vi "0716206_clock.vi"() -> ()   [LabVIEW 2021]
uses:
  <vilib>/Utility/miscctls.llb/LVPositionTypeDef.ctl
  <vilib>/Analysis/NI_AALBase.lvlib
panel:
  in  "Alarm Sound Path":path
  in  "Dial":dbl(knob) scale=0.0..1440.0
  in  "Set Time":bool
  out "Alarm Info.":string
  out "Sound Is Playing?":bool
  in  "Stop 2":bool
  in  "Sound Device ID":u32
  out "Alarm ring":bool=TRUE
  out "String 2":string
  out "String":string
  in  "Enable Alarm":bool
  in  "m0":bool
  in  "m1":bool
  in  "m2":bool
  in  "m3":bool
  in  "m4":bool
  in  "m5":bool
  out "alarm_min2":dbl
  in  "alarm_am":bool
  out "p.m.":bool
  out "alarm_min1":dbl
  out "alarm_hr":dbl
  in  "alarm_pm":bool
  in  "m2_1":bool
  in  "m2_2":bool
  in  "m2_3":bool
  in  "m2_4":bool
  in  "m2_5":bool
  in  "m2_6":bool
  in  "m2_7":bool
  in  "m2_8":bool
  in  "m2_9":bool
  in  "m2_0":bool
  out "P.M.":bool
  out "A.M.":bool
  in  "11":bool
  in  "1":bool
  in  "2":bool
  in  "3":bool
  in  "4":bool
  in  "5":bool
  in  "6":bool
  in  "7":bool
  in  "8":bool
  in  "9":bool
  in  "10":bool
  in  "0":bool
  in  "RESET":bool
  out "timer":dbl
  in  "PAUSE":bool
  in  "START":bool
  out "Clock":cluster{dbl[], dbl[]}[](graph)
  out "alarm picture":picture
  out "dial picture":picture
  # "12"
  # "set (custom time)"
  # "not set (system time)"
  # "3"
  # "9"
  # "6"
  # "disabled"
  # "enabled"
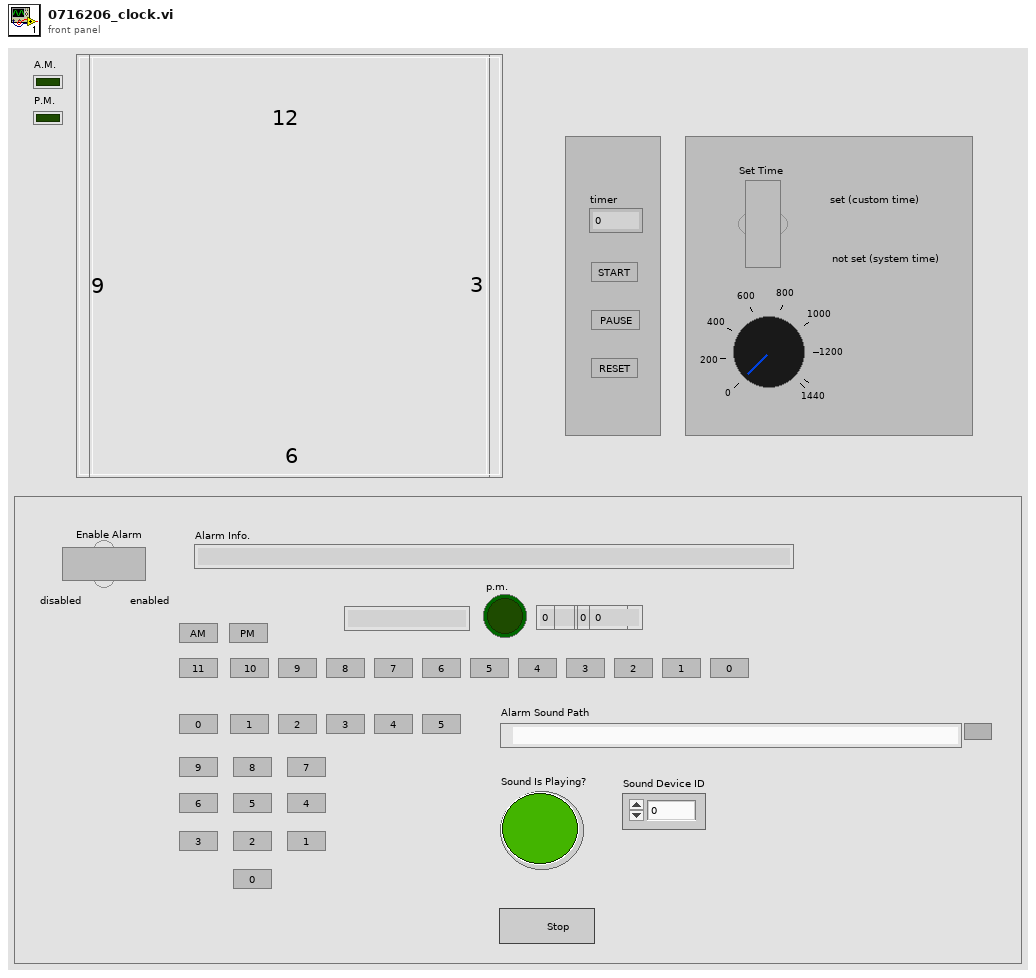
[diagram p1: front panel]
types:
  T1 = typedef "LVPositionTypeDef.ctl" = cluster{"Left":i32, "Top":i32}
  T2 = typedef "imagedata.ctl" = cluster{"image type":i32, "image depth":i32, "image":u8[], "mask":u8[], "colors":u32[], "Rectangle":cluster{"left":i16, "top":i16, "right":i16, "bottom":i16}}
  T3 = typedef "LVDateTimeRec.ctl" = cluster{"fractional second":dbl, "second":i32, "minute":i32, "hour":i32, "day of month":i32, "month":i32, "year":i32, "day of week":i32, "day of year":i32, "DST":i32}
  T4 = typedef "Sound Output Task ID.ctl" = u32
  T5 = cluster{"Sinusoidal Pattern":dbl[], "Sinusoidal Pattern":dbl[]}
  T6 = cluster{"Sinusoidal Pattern":dbl[], "Sinusoidal Pattern":dbl[]}[]
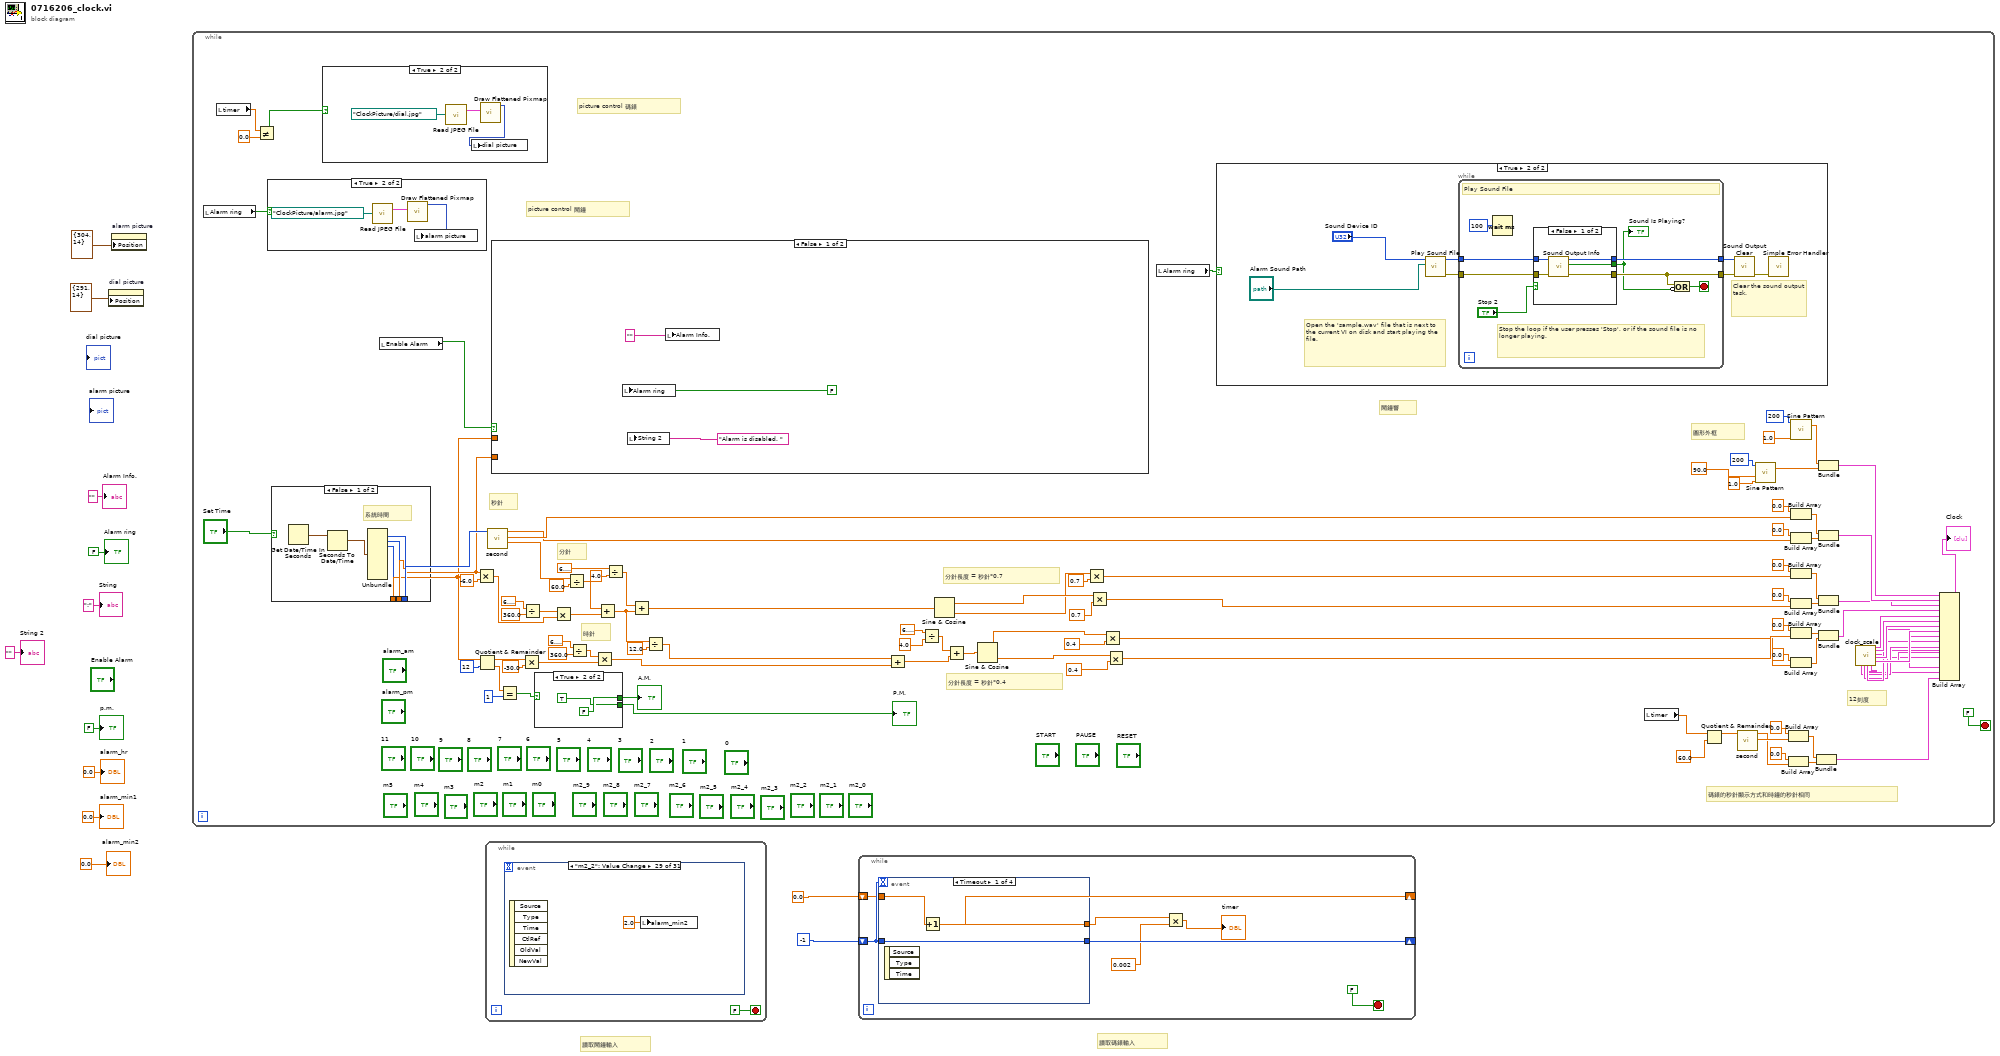
[diagram p0: block diagram]
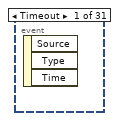
[diagram p2: hidden frame]
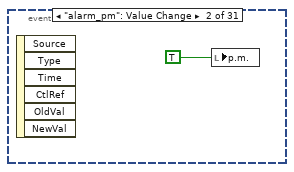
[diagram p3: hidden frame]
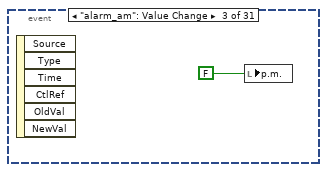
[diagram p4: hidden frame]
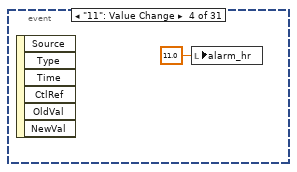
[diagram p5: hidden frame]
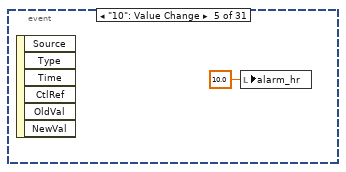
[diagram p6: hidden frame]
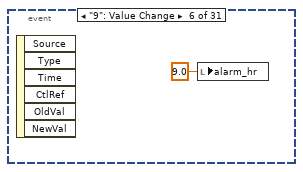
[diagram p7: hidden frame]
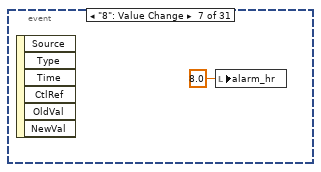
[diagram p8: hidden frame]
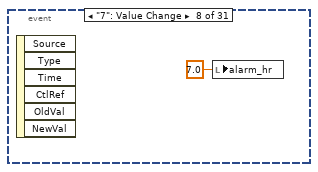
[diagram p9: hidden frame]
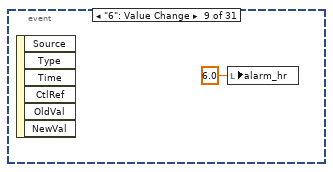
[diagram p10: hidden frame]
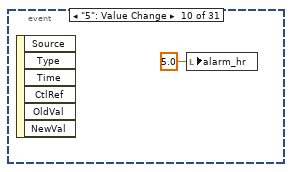
[diagram p11: hidden frame]
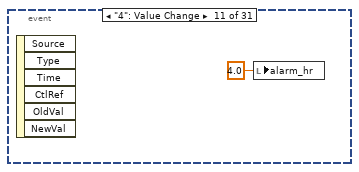
[diagram p12: hidden frame]
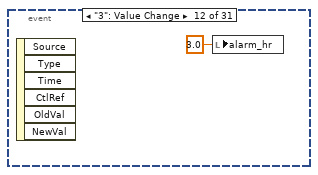
[diagram p13: hidden frame]
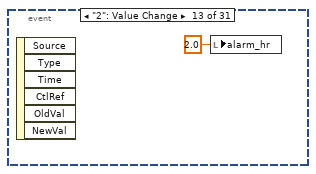
[diagram p14: hidden frame]
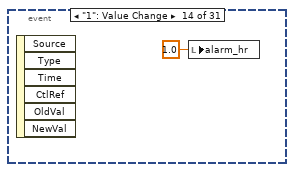
[diagram p15: hidden frame]
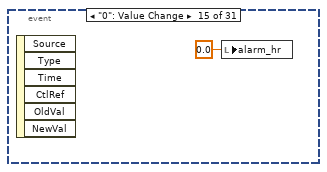
[diagram p16: hidden frame]
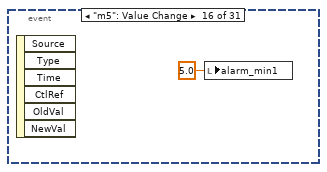
[diagram p17: hidden frame]
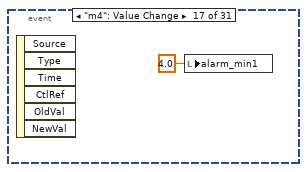
[diagram p18: hidden frame]
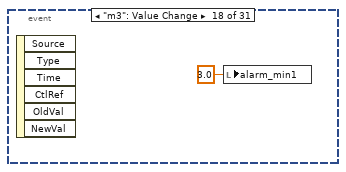
[diagram p19: hidden frame]
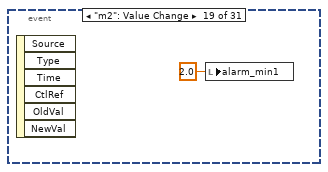
[diagram p20: hidden frame]
diagram:
  # "讀取碼錶輸入"
  # "讀取鬧鐘輸入"
  n1 = property on="dial picture" class="Pict"("Position"=T1 {"Left"=291, "Top"=14}) -> ()  [unwired: 2 in, 2 out]
  n2 = property on="alarm picture" class="Pict"("Position"=T1 {"Left"=304, "Top"=14}) -> ()  [unwired: 2 in, 2 out]
  n3 = while {
    stop <- FALSE stop-if-true
    # "picture control 鬧鐘"
    # "picture control 碼錶"
    # "鬧鐘響"
    # "碼錶的秒針顯示方式和時鐘的秒針相同"
    # "12刻度"
    # "圓形外框"
    # "分針長度 = 秒針*0.4"
    # "分針長度 = 秒針*0.7"
    # "時針"
    # "分針"
    # "秒針"
    n4 = local read "Alarm ring"() -> (w16:bool)
    n5 = local read "timer"() -> (w15:dbl)
    n6 = Not Equal?(x=w15, y=0.0) -> (x != y?=w13:bool)
    n7 = case shown="True" w16 {
      frame False {
        n8 = call "Empty Picture"() -> ("empty picture"=w122:picture)
        n9 = local write "alarm picture"(w122) -> ()
      }
      frame True {
        n10 = call <vilib>:"Read JPEG File.vi"("path to JPEG file"=path "ClockPicture/alarm.jpg" ("path to PNG file")) -> ("image data"=w125:T2)  [unwired: 8 in, 2 out]
        n11 = call <vilib>:"Draw Flattened Pixmap.vi"("image data"=w125) -> ("new picture"=w123:picture)  [unwired: 8 in]
        n12 = local write "alarm picture"(w123) -> ()
      }
    }
    n13 = case shown="False" "Set Time" {
      tunnel: [w129 w134] -> w19
      tunnel: [w128 w133] -> w18
      tunnel: [w127 w132] -> w17
      frame False {
        # "系統時間"
        n14 = Get Date/Time In Seconds() -> (seconds since 1Jan1904=w130:timestamp)
        n15 = Seconds To Date/Time(time stamp (now)=w130) -> (date time rec=w126:T3)  [unwired: 1 in]
        n16 = Unbundle(w126) -> ("second"=w129:i32, "minute"=w128:i32, "hour"=w127:i32)  [unwired: 7 out]
      }
      frame True {
        # "自訂時間"
        n17 = Get Date/Time In Seconds() -> (seconds since 1Jan1904=w137:timestamp)
        n18 = Seconds To Date/Time(time stamp (now)=w137) -> (date time rec=w131:T3)  [unwired: 1 in]
        n19 = Quotient & Remainder(x="Dial", y=60.0) -> (x-y*floor(x/y)=w133:dbl, floor(x/y)=w132:dbl)
        n20 = Unbundle(w131) -> ("second"=w134:i32)  [unwired: 9 out]
      }
    }
    n21 = case shown="True" w13 {
      frame False {
        n22 = call "Empty Picture"() -> ("empty picture"=w118:picture)
        n23 = local write "dial picture"(w118) -> ()
      }
      frame True {
        n24 = call <vilib>:"Read JPEG File.vi"("path to JPEG file"=path "ClockPicture/dial.jpg" ("path to PNG file")) -> ("image data"=w121:T2)  [unwired: 8 in, 2 out]
        n25 = call <vilib>:"Draw Flattened Pixmap.vi"("image data"=w121) -> ("new picture"=w119:picture)  [unwired: 8 in]
        n26 = local write "dial picture"(w119) -> ()
      }
    }
    n27 = local read "Enable Alarm"() -> (w22:bool)
    n28 = Multiply(x=w18, y=-6.0) -> (x*y=w106:dbl)
    n29 = Quotient & Remainder(x=w17, y=12) -> (x-y*floor(x/y)=w83:dbl, floor(x/y)=w27:dbl)
    n30 = call "second.vi"("second"=w19) -> ("Numeric"=w112:dbl, "Numeric 3"=w117:dbl, "Numeric 2"=w116:dbl)  [unwired: 8 in]
    n31 = case shown="False" w22 {
      tunnel: w18 -> [_ w178]
      tunnel: w17 -> [_ w177]
      frame False {
        n32 = local write "Alarm ring"(FALSE ("Alarm ring")) -> ()
        n33 = local write "String 2"("Alarm is disabled. " ("String 2")) -> ()
        n34 = local write "Alarm Info."("" ("Alarm Info.")) -> ()
      }
      frame True {
        # "鬧鐘分 = 鐘分"
        # "鬧鐘時 = 鐘時"
        n35 = local read "alarm_min1"() -> (w176:dbl)
        n36 = local read "alarm_hr"() -> (w167:dbl)
        n37 = local read "p.m."() -> (w168:bool)
        n38 = local read "alarm_min2"() -> (w173:dbl)
        n39 = case shown="True" w168 {
          tunnel: w167 -> [w180 w182]
          tunnel: [w180 w181] -> w166
          frame False {
          }
          frame True {
            n40 = Add(x=w182, y=12.0) -> (x+y=w181:dbl)
          }
        }
        n41 = Multiply(x=w176, y=10.0) -> (x*y=w174:dbl)
        n42 = Equal?(x=w166, y=w177) -> (x = y?=w170:bool)
        n43 = Add(x=w174, y=w173) -> (x+y=w172:dbl)
        n44 = Equal?(x=w172, y=w178) -> (x = y?=w171:bool)
        n45 = And(x=w171, y=w170) -> (x .and. y?=w169:bool)
        n46 = case shown="False" w169 {
          frame False {
            n47 = local write "Alarm ring"(FALSE ("Alarm ring")) -> ()
            n48 = local write "Alarm Info."("" ("Alarm Info.")) -> ()
          }
          frame True {
            n49 = local write "Alarm ring"(TRUE ("Alarm ring")) -> ()
            n50 = local write "Alarm Info."("Your alarm is ringing right now.  To stop and return to clock, first press 'Enable Alarm'  then press 'Stop'." ("Alarm Info.")) -> ()
          }
        }
        n51 = local write "String 2"("Alarm is set at " ("String 2")) -> ()
      }
    }
    n52 = Equal?(x=w27, y=1) -> (x = y?=w25:bool)
    n53 = Multiply(x=w83, y=-30.0) -> (x*y=w80:dbl)
    n54 = Divide(x=6.283185307179586, y=360.0) -> (x/y=w107:dbl)
    n55 = case shown="True" w25 {
      tunnel: [TRUE FALSE] -> w24
      tunnel: [FALSE TRUE] -> w23
      frame False {
      }
      frame True {
      }
    }
    "P.M." <- w23
    "A.M." <- w24
    n56 = Multiply(x=w107, y=w106) -> (x*y=w110:dbl)
    n57 = Divide(x=w112, y=60.0) -> (x/y=w111:dbl)
    n58 = Divide(x=6.283185307179586, y=360.0) -> (x/y=w79:dbl)
    n59 = Multiply(x=w79, y=w80) -> (x*y=w75:dbl)
    n60 = Add(x=w111, y=w110) -> (x+y=w77:dbl)
    n61 = Divide(x=6.283185307179586, y=4.0) -> (x/y=w102:dbl)
    n62 = Add(x=w102, y=w77) -> (x+y=w101:dbl)
    n63 = Divide(x=w77, y=12.0) -> (x/y=w76:dbl)
    n64 = Add(x=w76, y=w75) -> (x+y=w71:dbl)
    n65 = Divide(x=6.283185307179586, y=4.0) -> (x/y=w72:dbl)
    n66 = Sine & Cosine(0:w101) -> (1:w98:dbl, 2:w97:dbl)
    n67 = Add(x=w72, y=w71) -> (x+y=w70:dbl)
    n68 = Sine & Cosine(0:w70) -> (1:w62:dbl, 2:w61:dbl)
    n69 = Multiply(x=w97, y=0.7) -> (x*y=w95:dbl)
    n70 = Multiply(x=w98, y=0.7) -> (x*y=w96:dbl)
    n71 = Multiply(x=w62, y=0.4) -> (x*y=w59:dbl)
    n72 = Multiply(x=w61, y=0.4) -> (x*y=w60:dbl)
    n73 = local read "Alarm ring"() -> (w21:bool)
    n74 = case shown="True" w21 {
      frame False {
      }
      frame True {
        # "Clear the sound output task."
        # "Open the 'sample.wav' file that is next to the current VI on disk and start playing the file."
        n75 = call <vilib>:"Play Sound File.vi"("path"="Alarm Sound Path", "device ID"="Sound Device ID") -> ("error out"=w140:errorcluster, "task ID"=w139:T4)  [unwired: 8 in]
        n76 = while {
          tunnel: w139 -> [w146]
          tunnel: [w151] -> w142
          tunnel: w140 -> [w147]
          tunnel: [w150] -> w141
          stop <- w152 stop-if-true
          # "Stop the loop if the user presses 'Stop', or if the sound file is no longer playing."
          # "Play Sound File"
          n77 = Wait (ms)(milliseconds to wait=u32 100) -> ()  [unwired: 1 out]
          n78 = case shown="False" "Stop 2" {
            tunnel: w147 -> [w157 w161]
            tunnel: [w156 w159] -> w151
            tunnel: w146 -> [w155 w162]
            tunnel: [w154 w160] -> w150
            tunnel: [w153 FALSE] -> w149
            frame False {
              n79 = call <vilib>:"Sound Output Info.vi"("error in (no error)"=w157, "task ID"=w155) -> ("error out"=w154:errorcluster, "is playing?"=w153:bool, "task ID out"=w156:T4)  [unwired: 6 in, 1 out]
            }
            frame True {
              n80 = call <vilib>:"Sound Output Stop.vi"("error in (no error)"=w161, "task ID"=w162) -> ("error out"=w160:errorcluster, "task ID out"=w159:T4)  [unwired: 8 in]
            }
          }
          "Sound Is Playing?" <- w149
          n81 = Compound Arithmetic op=OR(w150, invert w149) -> (w152:bool)
        }
        n82 = call <vilib>:"Sound Output Clear.vi"("error in (no error)"=w141, "task ID"=w142) -> ("error out"=w144:errorcluster)  [unwired: 9 in]
        n83 = call <vilib>:"Simple Error Handler.vi"("error in (no error)"=w144) -> ()  [unwired: 4 in, 5 out]
      }
    }
    n84 = local read "timer"() -> (w32:dbl)
    n85 = Quotient & Remainder(x=w32, y=60.0) -> (x-y*floor(x/y)=w31:dbl)  [unwired: 1 out]
    n86 = call "second.vi"("second"=w31) -> ("Numeric 3"=w30:dbl, "Numeric 2"=w29:dbl)  [unwired: 8 in, 1 out]
    n87 = call <vilib>:"Sine Pattern.vi"("cycles"=1.0, "phase(degrees)"=90.0, "samples"=200) -> ("Sinusoidal Pattern"=w53:dbl[])  [unwired: 1 in, 1 out]
    n88 = Build Array(0.0, w30) -> (w36:dbl[])
    n89 = Build Array(0.0, w29) -> (w35:dbl[])
    n90 = call <vilib>:"Sine Pattern.vi"("cycles"=1.0, "samples"=200) -> ("Sinusoidal Pattern"=w54:dbl[])  [unwired: 2 in, 1 out]
    n91 = Build Array(0.0 ("element"), w117) -> (w88:dbl[])
    n92 = Build Array(0.0 ("element"), w116) -> (w89:dbl[])
    n93 = Build Array(0.0 ("element"), w95) -> (w91:dbl[])
    n94 = Build Array(0.0 ("element"), w96) -> (w92:dbl[])
    n95 = Build Array(0.0 ("element"), w60) -> (w64:dbl[])
    n96 = Build Array(0.0 ("element"), w59) -> (w65:dbl[])
    n97 = Bundle(w36, w35) -> (w34:cluster{dbl[], dbl[]})  [unwired: 1 in]
    n98 = Bundle("Sinusoidal Pattern"=w54, "Sinusoidal Pattern"=w53) -> (w51:T5)  [unwired: 1 in]
    n99 = Bundle(w88, w89) -> (w115:cluster{dbl[], dbl[]})  [unwired: 1 in]
    n100 = Bundle(w91, w92) -> (w90:cluster{dbl[], dbl[]})  [unwired: 1 in]
    n101 = Bundle(w64, w65) -> (w63:cluster{dbl[], dbl[]})  [unwired: 1 in]
    n102 = call "clock_scale.vi"() -> ("Cluster 6"=w44:cluster{dbl[], dbl[]}, "Cluster 3"=w41:cluster{dbl[], dbl[]}, "Cluster 7"=w45:cluster{dbl[], dbl[]}, "Cluster 2"=w40:cluster{dbl[], dbl[]}, "Cluster 8"=w46:cluster{dbl[], dbl[]}, "Cluster"=w39:cluster{dbl[], dbl[]}, "Cluster 9"=w47:cluster{dbl[], dbl[]}, "Cluster 12"=w50:cluster{dbl[], dbl[]}, "Cluster 11"=w49:cluster{dbl[], dbl[]}, "Cluster 4"=w42:cluster{dbl[], dbl[]}, "Cluster 10"=w48:cluster{dbl[], dbl[]}, "Cluster 5"=w43:cluster{dbl[], dbl[]})  [unwired: 8 in]
    n103 = Build Array(w51, w115, w90, w63, w50, w49, w48, w47, w46, w45, w44, w43, w42, w41, w40, w39, w34) -> (→"Clock":T6)
  }
  n104 = while {
    stop <- FALSE stop-if-true
    n105 = event shown="[28] \"m2_2\": Value Change" {
      selector: _ -> [_ _ _ _ _ _ _ _ _ _ _ _ _ _ _ _ _ _ _ _ _ _ _ _ _ _ _ _ _ _ _]
      dyn-events: _ -> [_ _ _ _ _ _ _ _ _ _ _ _ _ _ _ _ _ _ _ _ _ _ _ _ _ _ _ _ _ _ _]
      timeout: _ -> [_ _ _ _ _ _ _ _ _ _ _ _ _ _ _ _ _ _ _ _ _ _ _ _ _ _ _ _ _ _ _]
      event Timeout {
        n106 = event-data() -> ()  [unwired: 1 in, 3 out]
      }
      event "alarm_pm": Value Change {
        n107 = event-data() -> ()  [unwired: 1 in, 6 out]
        n108 = local write "p.m."(TRUE ("alarm_is_pm")) -> ()
      }
      event "alarm_am": Value Change {
        n109 = event-data() -> ()  [unwired: 1 in, 6 out]
        n110 = local write "p.m."(FALSE ("alarm_is_pm")) -> ()
      }
      event "11": Value Change {
        n111 = event-data() -> ()  [unwired: 1 in, 6 out]
        n112 = local write "alarm_hr"(11.0 ("alarm_hr")) -> ()
      }
      event "10": Value Change {
        n113 = event-data() -> ()  [unwired: 1 in, 6 out]
        n114 = local write "alarm_hr"(10.0 ("alarm_hr")) -> ()
      }
      event "9": Value Change {
        n115 = event-data() -> ()  [unwired: 1 in, 6 out]
        n116 = local write "alarm_hr"(9.0 ("alarm_hr")) -> ()
      }
      event "8": Value Change {
        n117 = event-data() -> ()  [unwired: 1 in, 6 out]
        n118 = local write "alarm_hr"(8.0 ("alarm_hr")) -> ()
      }
      event "7": Value Change {
        n119 = event-data() -> ()  [unwired: 1 in, 6 out]
        n120 = local write "alarm_hr"(7.0 ("alarm_hr")) -> ()
      }
      event "6": Value Change {
        n121 = event-data() -> ()  [unwired: 1 in, 6 out]
        n122 = local write "alarm_hr"(6.0 ("alarm_hr")) -> ()
      }
      event "5": Value Change {
        n123 = event-data() -> ()  [unwired: 1 in, 6 out]
        n124 = local write "alarm_hr"(5.0 ("alarm_hr")) -> ()
      }
      event "4": Value Change {
        n125 = event-data() -> ()  [unwired: 1 in, 6 out]
        n126 = local write "alarm_hr"(4.0 ("alarm_hr")) -> ()
      }
      event "3": Value Change {
        n127 = event-data() -> ()  [unwired: 1 in, 6 out]
        n128 = local write "alarm_hr"(3.0 ("alarm_hr")) -> ()
      }
      event "2": Value Change {
        n129 = event-data() -> ()  [unwired: 1 in, 6 out]
        n130 = local write "alarm_hr"(2.0 ("alarm_hr")) -> ()
      }
      event "1": Value Change {
        n131 = event-data() -> ()  [unwired: 1 in, 6 out]
        n132 = local write "alarm_hr"(1.0 ("alarm_hr")) -> ()
      }
      event "0": Value Change {
        n133 = event-data() -> ()  [unwired: 1 in, 6 out]
        n134 = local write "alarm_hr"(0.0 ("alarm_hr")) -> ()
      }
      event "m5": Value Change {
        n135 = event-data() -> ()  [unwired: 1 in, 6 out]
        n136 = local write "alarm_min1"(5.0 ("alarm_min1")) -> ()
      }
      event "m4": Value Change {
        n137 = event-data() -> ()  [unwired: 1 in, 6 out]
        n138 = local write "alarm_min1"(4.0 ("alarm_min1")) -> ()
      }
      event "m3": Value Change {
        n139 = event-data() -> ()  [unwired: 1 in, 6 out]
        n140 = local write "alarm_min1"(3.0 ("alarm_min1")) -> ()
      }
      event "m2": Value Change {
        n141 = event-data() -> ()  [unwired: 1 in, 6 out]
        n142 = local write "alarm_min1"(2.0 ("alarm_min1")) -> ()
      }
      event "m1": Value Change {
        n143 = event-data() -> ()  [unwired: 1 in, 6 out]
        n144 = local write "alarm_min1"(1.0 ("alarm_min1")) -> ()
      }
      event "m0": Value Change {
        n145 = event-data() -> ()  [unwired: 1 in, 6 out]
        n146 = local write "alarm_min1"(0.0 ("alarm_min1")) -> ()
      }
      event "m2_9": Value Change {
        n147 = event-data() -> ()  [unwired: 1 in, 6 out]
        n148 = local write "alarm_min2"(9.0 ("alarm_min2")) -> ()
      }
      event "m2_8": Value Change {
        n149 = event-data() -> ()  [unwired: 1 in, 6 out]
        n150 = local write "alarm_min2"(8.0 ("alarm_min2")) -> ()
      }
      event "m2_7": Value Change {
        n151 = event-data() -> ()  [unwired: 1 in, 6 out]
        n152 = local write "alarm_min2"(7.0 ("alarm_min2")) -> ()
      }
      event "m2_6": Value Change {
        n153 = event-data() -> ()  [unwired: 1 in, 6 out]
        n154 = local write "alarm_min2"(6.0 ("alarm_min2")) -> ()
      }
      event "m2_5": Value Change {
        n155 = event-data() -> ()  [unwired: 1 in, 6 out]
        n156 = local write "alarm_min2"(5.0 ("alarm_min2")) -> ()
      }
      event "m2_4": Value Change {
        n157 = event-data() -> ()  [unwired: 1 in, 6 out]
        n158 = local write "alarm_min2"(4.0 ("alarm_min2")) -> ()
      }
      event "m2_3": Value Change {
        n159 = event-data() -> ()  [unwired: 1 in, 6 out]
        n160 = local write "alarm_min2"(3.0 ("alarm_min2")) -> ()
      }
      event "m2_2": Value Change {
        n161 = event-data() -> ()  [unwired: 1 in, 6 out]
        n162 = local write "alarm_min2"(2.0 ("alarm_min2")) -> ()
      }
      event "m2_1": Value Change {
        n163 = event-data() -> ()  [unwired: 1 in, 6 out]
        n164 = local write "alarm_min2"(1.0 ("alarm_min2")) -> ()
      }
      event "m2_0": Value Change {
        n165 = event-data() -> ()  [unwired: 1 in, 6 out]
        n166 = local write "alarm_min2"(0.0 ("alarm_min2")) -> ()
      }
    }
  }
  n167 = while {
    shift-right: [w229] -> _
    shift-left: -1 -> [w228]
    shift-right: [w225] -> _
    shift-left: 0.0 -> [w226]
    stop <- FALSE stop-if-true
    n168 = event shown="[0] Timeout" {
      selector: _ -> [_ _ _ _]
      dyn-events: _ -> [_ _ _ _]
      timeout: w228 -> [_ _ _ _]
      tunnel: [w232 1 -1 -1] -> w229
      tunnel: w228 -> [w232 _ _ _]
      tunnel: w226 -> [w231 w233 w235 _]
      tunnel: [w230 w233 w235 0.0] -> w225
      event Timeout {
        n169 = event-data() -> ()  [unwired: 1 in, 3 out]
        n170 = Increment(x=w231) -> (x+1=w230:dbl)
      }
      event "START": Value Change {
        n171 = event-data() -> ()  [unwired: 1 in, 4 out]
      }
      event "PAUSE": Value Change {
        n172 = event-data() -> ()  [unwired: 1 in, 4 out]
      }
      event "RESET": Value Change {
        n173 = event-data() -> ()  [unwired: 1 in, 4 out]
      }
    }
    n174 = Multiply(x=w225, y=0.002) -> (x*y=→"timer":dbl)
  }
  "alarm_hr" <- 0.0 ("alarm_hr")
  "alarm_min1" <- 0.0 ("alarm_min")
  "p.m." <- FALSE ("alarm_is_pm")
  "alarm_min2" <- 0.0 ("alarm_min2")
  "String" <- ":" ("String")
  "String 2" <- "" ("String 2")
  "Alarm ring" <- FALSE ("Alarm ring")
  "Alarm Info." <- ""
